vi "Insight_RW_Delay.vi"(6 "Major Version":i32, 7 "Parameter Type":enum16{"Value", "MAXimum", "MINimum", "DEFault"}(ring), 8 "error in (no error)":errorcluster, 9 "Mode (Read / Write)":enum8{"Write", "Read"}(ring), 10 "Intersweep Delay (ns)":dbl=100.0, 11 "telnet connection":T1) -> (0 "error out":errorcluster, 1 "response data":string, 2 "Intersweep Delay (ns)":dbl format="%.4g", 3 "telnet  connection out":T1)   [LabVIEW 2015]
doc: "Insight Photonic Solutions\n\nInsight Photonic Solutions\n\nThis VI reads or writes the Duty Cycle of the laser sweep.\n\nINPUTS\n\nMode - Tells the VI whether the command is a Read or a Write. (Default = Read).\nParameter Type - Tells the VI whether the command should use a Value or a keyword MAXimum, MINimum or DEFault to set the parameter value. (Default = Value).\nDuty Cycle (%) - The numeric value to set the Duty Cycle of a sweep. (Default = 100).\nerror in - The standard LabView Error cluster. Use this to enforce sequentiality and error tracking.\n\nOUTPUTS\n\nresponse data - the complete response string from the laser\nDuty Cycle (%)? - the Duty Cycle of the sweep that is written to or read from the laser\nerror out - the standard error cluster. Reports errors in reading or writing to the laser, or passes through errors from before this VI.\n\nver 1.0 - original release"
uses:
  Telnet Session.ctl
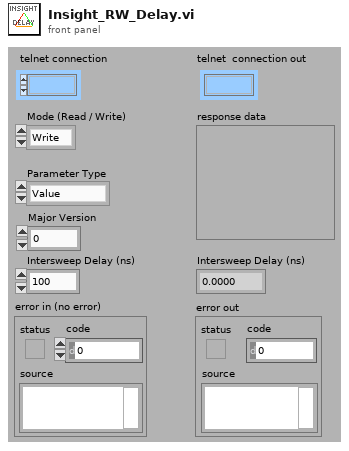
[diagram p1: front panel]
types:
  T1 = typedef "Telnet Session.ctl" = refnum<k1>
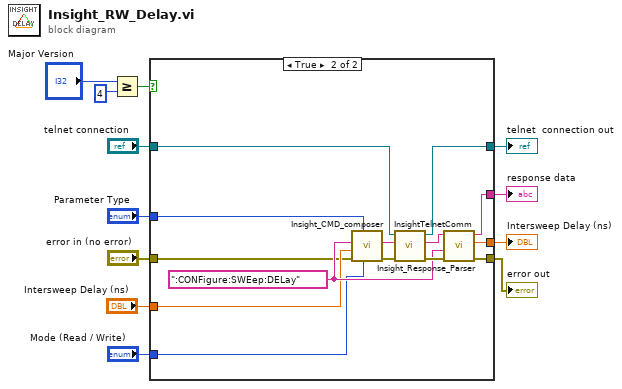
[diagram p0: block diagram]
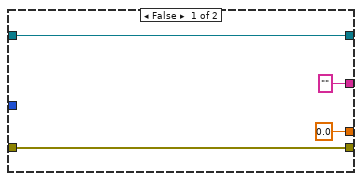
[diagram p2: hidden frame]
diagram:
  n1 = Greater Or Equal?(x="Major Version", y=4) -> (x >= y?=w1:bool)
  n2 = case shown="True" w1 {
    tunnel: "telnet connection" -> [w13 w25]
    tunnel: "Parameter Type" -> [_ w24]
    tunnel: "Intersweep Delay (ns)" -> [_ w23]
    tunnel: "error in (no error)" -> [w15 w22]
    tunnel: "Mode (Read / Write)" -> [_ w21]
    tunnel: [w13 w20] -> w7
    tunnel: ["" ("Laser Response Out") w19] -> w6
    tunnel: [0.0 ("Value") w18] -> w5
    tunnel: [w15 w17] -> w4
    frame False {
    }
    frame True {
      w27 = ":CONFigure:SWEep:DELay" ("String")
      n3 = call "Insight_CMD_composer.vi"("Mode (Read / Write)"=w21, "Parameter Type"=w24, "error in (no error)"=w22, "Value"=w23, "CMD"=w27) -> ("error out"=w30:errorcluster, "Command String"=w29:string)  [unwired: 5 in]
      n4 = call "InsightTelnetComm.vi"("error in"=w30, "write buffer (\"\")"=w29, "telnet connection"=w25) -> ("error out"=w28:errorcluster, "response data"=w26:string, "telnet  connection out"=w20:T1)  [unwired: 4 in]
      n5 = call "Insight_Response_Parser.vi"("error in (no error)"=w28, "Command String"=w27, "Laser Response In"=w26) -> ("error out"=w17:errorcluster, "Value"=w18:dbl, "Laser Response Out"=w19:string)  [unwired: 6 in]
    }
  }
  "Intersweep Delay (ns)" <- w5
  "response data" <- w6
  "telnet  connection out" <- w7
  "error out" <- w4
